vi "TPG361_Status.vi"() -> (1 "n_ng":u8, 2 "values":cluster{"TPG361_ST":u32, "TPG361_p":dbl})   [LabVIEW 2019]
uses:
  TPG361_Global.vi
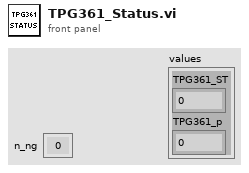
[diagram p1: front panel]
types:
  T1 = enum32{"Bad", "Idle", "Run top level", "Running"}
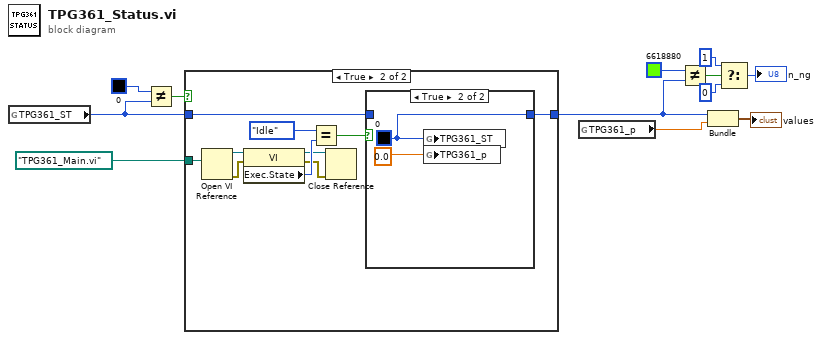
[diagram p0: block diagram]
diagram:
  n1 = global read "TPG361_Global.vi" "TPG361_ST"() -> (w3:u32)
  n2 = Not Equal?(x=u32 0 ("MKS670_1000_ST 2"), y=w3) -> (x != y?=w12:bool)
  n3 = case shown="True" w12 {
    tunnel: w3 -> [w13 w15]
    tunnel: [w13 w14] -> w9
    tunnel: path "TPG361_Main.vi" ("vi path") -> [_ w16]
    frame False {
    }
    frame True {
      n4 = Open VI Reference(vi path=w16) -> (vi reference=w23:refnum<vi>, error out=w22:errorcluster)  [unwired: 5 in]
      n5 = property class="VI"(reference=w23, error in=w22) -> (reference out=w18:refnum<vi>, error out=w17:errorcluster, "Exec.State"=w20:T1)
      n6 = Equal?(x=T1."Idle" ("Execution:State"), y=w20) -> (x = y?=w21:bool)
      n7 = Close Reference(reference=w18, error in (no error)=w17) -> ()  [unwired: 1 out]
      n8 = case shown="True" w21 {
        tunnel: w15 -> [w24 _]
        tunnel: [w24 w26] -> w14
        frame False {
        }
        frame True {
          w26 = u32 0 ("MKS670_1000_ST")
          n9 = global write "TPG361_Global.vi" "TPG361_ST"(w26) -> ()
          n10 = global write "TPG361_Global.vi" "TPG361_p"(0.0 ("MKS670_1000_P")) -> ()
        }
      }
    }
  }
  n11 = global read "TPG361_Global.vi" "TPG361_p"() -> (w2:dbl)
  n12 = Not Equal?(x=u32 6618880 ("MKS670_1000_ST 2"), y=w9) -> (x != y?=w7:bool)
  n13 = Bundle("MKS670_1000_ST"=w9, "TPG361_p"=w2) -> (→"values":cluster{"MKS670_1000_ST":u32, "TPG361_p":dbl})  [unwired: 1 in]
  n14 = Select(t=u8 1 ("n_ng"), s=w7, f=u8 0 ("n_ng")) -> (s? t:f=→"n_ng":u8)
